vi "WS1050 VPI Test.vi"(0 "Ke2000 Input":refnum<visa-resource-name>, 1 "AD7747 In":refnum<visa-resource-name>, 3 "RFFE In":refnum<visa-resource-name>, 4 "Command":string[](array[string])=["074100", "07413B", "07423B", "07433B", "07413B", "074100"], 5 "CP Control":string, 7 "error out":errorcluster, 8 "Sequence Names":string[](array[string])=["CMin_35V", "C1L_35V", "C2L_35V", "C3L_35V", "ALL_ON_35V", "ALL_OFF_35V"], 9 "S_ValueC1(pF)":dbl=-4.5642919921875, 11 "S_ValueC3(pF)":dbl=-4.9974111328125, 12 "Delay Cap Meas":u32, 13 "S_ValueC2(pF)":dbl=-4.9191376953125, 14 "Status In":string="Idle.....", 17 "VPI Voltage":string) -> (16 "Data Out":string[](array[string]), 20 "Ke2000 Output":refnum<visa-resource-name>, 21 "AD7747 Out":refnum<visa-resource-name>, 23 "RFFE Out":refnum<visa-resource-name>, 24 "Status":string="Idle.....", 25 "IDD_VPI ON":string="43.552393E+0", 26 "IDD_VPI OFF":string="43.360206E+0", 27 "error out 2":errorcluster)   [LabVIEW 2017]
panel:
  out "Sequence":i32(listbox)=5
  out "CMin2_35V":string[](array[string])=["1.184179E+0", "1.241177E+0", "1.250951E+0"]
  out "Cmax 35V":string[](array[string])=["7.353896E+0", "7.168632E+0", "7.184664E+0"]
  out "C3L_Max 35V":string="7.184664E+0"
  out "C2L_Max 35V":string="7.168632E+0"
  out "C1L_Max 35V":string="7.353896E+0"
  out "CMin_35V":string[](array[string])=["1.183737E+0", "1.240778E+0", "1.250697E+0"]
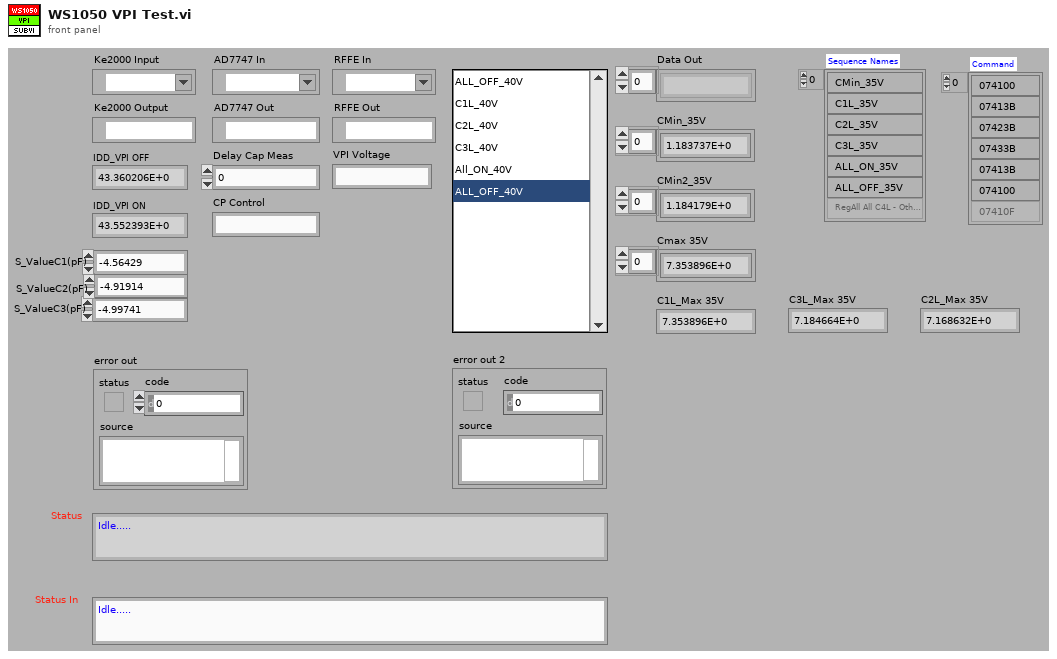
[diagram p1: front panel]
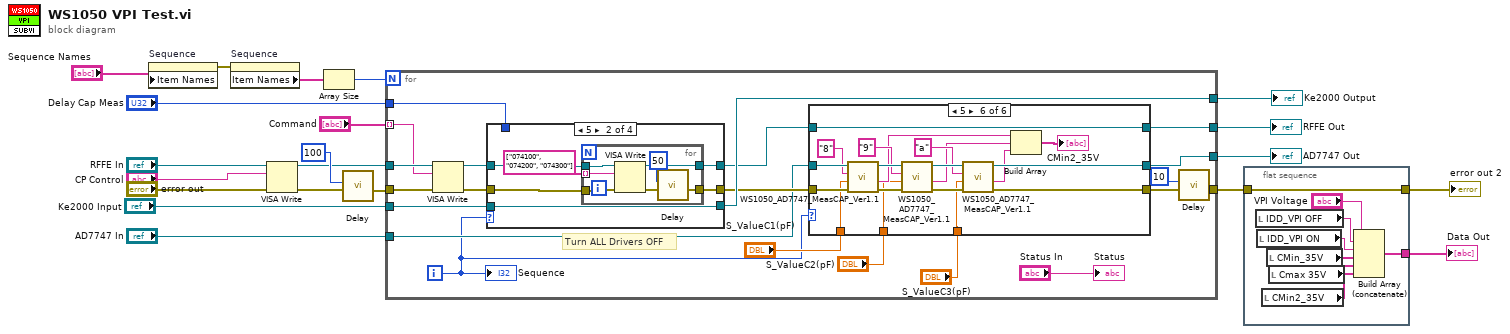
[diagram p0: block diagram]
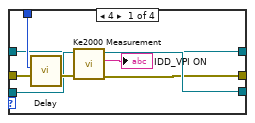
[diagram p2: hidden frame]
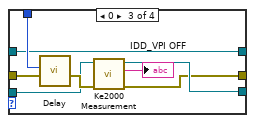
[diagram p3: hidden frame]
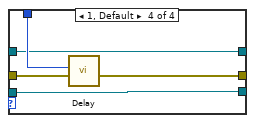
[diagram p4: hidden frame]
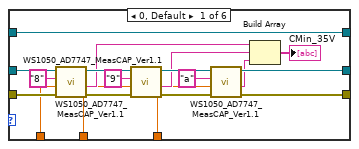
[diagram p5: hidden frame]
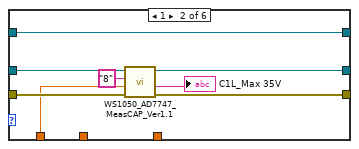
[diagram p6: hidden frame]
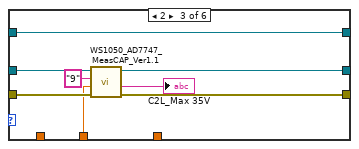
[diagram p7: hidden frame]
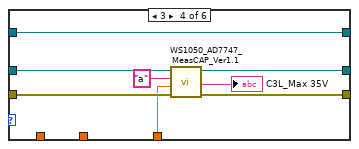
[diagram p8: hidden frame]
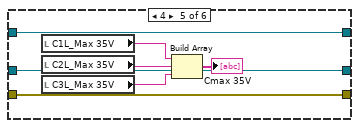
[diagram p9: hidden frame]
diagram:
  n1 = property on="Sequence" class="LstBox (strict)"("Item Names"="Sequence Names") -> (error out=w16:errorcluster)  [unwired: 2 in, 1 out]
  n2 = property on="Sequence" class="LstBox (strict)"(error in=w16) -> ("Item Names"=w14:string[])  [unwired: 1 in, 2 out]
  n3 = VISA Write(VISA resource name="RFFE In", write buffer="CP Control", error in (no error)="error out") -> (VISA resource name out=w11:refnum<visa-resource-name>, error out=w1:errorcluster)  [unwired: 1 out]
  n4 = Array Size(array=w14) -> (size(s)=w17:i32)
  n5 = call "Delay.vi"("error in (no error)"=w1, "milliseconds to wait"=u32 100) -> ("error out"=w2:errorcluster)  [unwired: 9 in]
  n6 = for {
    N: w17 -> [_]
    tunnel: [w28] -> w10
    tunnel: [w34] -> w5
    tunnel: "Delay Cap Meas" -> [w42]
    tunnel: w2 -> [w38]
    tunnel: "Ke2000 Input" -> [w41]
    tunnel: w11 -> [w40]
    tunnel: "Command" -> [w39] mode=indexing
    tunnel: [w36] -> w9
    tunnel: "AD7747 In" -> [w32]
    tunnel: [w30] -> w6
    i -> [w23]
    # "Turn ALL Drivers OFF"
    n7 = VISA Write(VISA resource name=w40, write buffer=w39, error in (no error)=w38) -> (VISA resource name out=w35:refnum<visa-resource-name>, error out=w37:errorcluster)  [unwired: 1 out]
    n8 = case shown="5" w23 {
      tunnel: [w44 w55 w65 w76] -> w33
      tunnel: w42 -> [w46 _ w67 w75]
      tunnel: [w49 w51 w70 w73] -> w36
      tunnel: w37 -> [w47 w56 w68 w74]
      tunnel: w41 -> [w45 w51 w66 w73]
      tunnel: w35 -> [w43 w53 w64 w72]
      tunnel: [w43 w52 w64 w72] -> w31
      frame 4 {
        n9 = call "Delay.vi"("error in (no error)"=w47, "milliseconds to wait"=w46) -> ("error out"=w48:errorcluster)  [unwired: 9 in]
        n10 = call "Ke2000 Measurement.vi"("error in (no error)"=w48, "VISA resource name"=w45) -> ("error out"=w44:errorcluster, "Meas in micro"=→"IDD_VPI ON":string, "VISA resource name out"=w49:refnum<visa-resource-name>)  [unwired: 4 in, 3 out]
      }
      frame 5 {
        n11 = for {
          tunnel: w56 -> [w63]
          tunnel: [w60] -> w55
          tunnel: [w59] -> w52
          tunnel: w53 -> [w58]
          tunnel: string[] ["074100", "074200", "074300"] -> [w57] mode=indexing
          n12 = VISA Write(VISA resource name=w58, write buffer=w57, error in (no error)=w63) -> (VISA resource name out=w59:refnum<visa-resource-name>, error out=w62:errorcluster)  [unwired: 1 out]
          n13 = call "Delay.vi"("error in (no error)"=w62, "milliseconds to wait"=u32 50) -> ("error out"=w60:errorcluster)  [unwired: 9 in]
        }
      }
      frame 0 {
        n14 = call "Delay.vi"("error in (no error)"=w68, "milliseconds to wait"=w67) -> ("error out"=w69:errorcluster)  [unwired: 9 in]
        n15 = call "Ke2000 Measurement.vi"("error in (no error)"=w69, "VISA resource name"=w66) -> ("error out"=w65:errorcluster, "Meas in micro"=→"IDD_VPI OFF":string, "VISA resource name out"=w70:refnum<visa-resource-name>)  [unwired: 4 in, 3 out]
      }
      frame 1, Default {
        n16 = call "Delay.vi"("error in (no error)"=w74, "milliseconds to wait"=w75) -> ("error out"=w76:errorcluster)  [unwired: 9 in]
      }
    }
    n17 = case shown="5" w23 {
      tunnel: w32 -> [w94 w100 w108 w116 w126 w144]
      tunnel: [w85 w102 w110 w118 w125 w135] -> w29
      tunnel: w33 -> [w92 w103 w111 w119 w125 w142]
      tunnel: [w84 w99 w107 w115 w126 w136] -> w34
      tunnel: w31 -> [w80 w97 w105 w113 w124 w130]
      tunnel: [w80 w97 w105 w113 w124 w130] -> w30
      tunnel: "S_ValueC1(pF)" -> [w79 w96 _ _ _ w129]
      tunnel: "S_ValueC2(pF)" -> [w78 _ w104 _ _ w128]
      tunnel: "S_ValueC3(pF)" -> [w77 _ _ w112 _ w127]
      frame 0, Default {
        n18 = call "WS1050_AD7747_MeasCAP_Ver1.1.vi"("error in (no error)"=w92, "OFFSet Cal"=w79, "AD7747_Number"="8", "Control"=w94) -> ("error"=w95:errorcluster, "CAP (pF)"=w83:string, "Control out"=w93:refnum<visa-resource-name>)  [unwired: 3 in, 2 out]
        n19 = call "WS1050_AD7747_MeasCAP_Ver1.1.vi"("error in (no error)"=w95, "OFFSet Cal"=w78, "AD7747_Number"="9", "Control"=w93) -> ("error"=w91:errorcluster, "CAP (pF)"=w82:string, "Control out"=w89:refnum<visa-resource-name>)  [unwired: 3 in, 2 out]
        n20 = call "WS1050_AD7747_MeasCAP_Ver1.1.vi"("error in (no error)"=w91, "OFFSet Cal"=w77, "AD7747_Number"="a", "Control"=w89) -> ("error"=w85:errorcluster, "CAP (pF)"=w81:string, "Control out"=w84:refnum<visa-resource-name>)  [unwired: 3 in, 2 out]
        n21 = Build Array(w83, w82, w81) -> (→"CMin_35V":string[])
      }
      frame 1 {
        n22 = call "WS1050_AD7747_MeasCAP_Ver1.1.vi"("error in (no error)"=w103, "OFFSet Cal"=w96, "AD7747_Number"="8", "Control"=w100) -> ("error"=w102:errorcluster, "CAP (pF)"=→"C1L_Max 35V":string, "Control out"=w99:refnum<visa-resource-name>)  [unwired: 3 in, 2 out]
      }
      frame 2 {
        n23 = call "WS1050_AD7747_MeasCAP_Ver1.1.vi"("error in (no error)"=w111, "OFFSet Cal"=w104, "AD7747_Number"="9", "Control"=w108) -> ("error"=w110:errorcluster, "CAP (pF)"=→"C2L_Max 35V":string, "Control out"=w107:refnum<visa-resource-name>)  [unwired: 3 in, 2 out]
      }
      frame 3 {
        n24 = call "WS1050_AD7747_MeasCAP_Ver1.1.vi"("error in (no error)"=w119, "OFFSet Cal"=w112, "AD7747_Number"="a", "Control"=w116) -> ("error"=w118:errorcluster, "CAP (pF)"=→"C3L_Max 35V":string, "Control out"=w115:refnum<visa-resource-name>)  [unwired: 3 in, 2 out]
      }
      frame 4 {
        n25 = local read "C1L_Max 35V"() -> (w123:string)
        n26 = local read "C2L_Max 35V"() -> (w122:string)
        n27 = local read "C3L_Max 35V"() -> (w121:string)
        n28 = Build Array(w123, w122, w121) -> (→"Cmax 35V":string[])
      }
      frame 5 {
        n29 = call "WS1050_AD7747_MeasCAP_Ver1.1.vi"("error in (no error)"=w142, "OFFSet Cal"=w129, "AD7747_Number"="8", "Control"=w144) -> ("error"=w145:errorcluster, "CAP (pF)"=w133:string, "Control out"=w143:refnum<visa-resource-name>)  [unwired: 3 in, 2 out]
        n30 = call "WS1050_AD7747_MeasCAP_Ver1.1.vi"("error in (no error)"=w145, "OFFSet Cal"=w128, "AD7747_Number"="9", "Control"=w143) -> ("error"=w141:errorcluster, "CAP (pF)"=w132:string, "Control out"=w139:refnum<visa-resource-name>)  [unwired: 3 in, 2 out]
        n31 = call "WS1050_AD7747_MeasCAP_Ver1.1.vi"("error in (no error)"=w141, "OFFSet Cal"=w127, "AD7747_Number"="a", "Control"=w139) -> ("error"=w135:errorcluster, "CAP (pF)"=w131:string, "Control out"=w136:refnum<visa-resource-name>)  [unwired: 3 in, 2 out]
        n32 = Build Array(w133, w132, w131) -> (→"CMin2_35V":string[])
      }
    }
    n33 = call "Delay.vi"("error in (no error)"=w29, "milliseconds to wait"=u32 10) -> ("error out"=w28:errorcluster)  [unwired: 9 in]
    "Sequence" <- w23
    "Status" <- "Status In"
  }
  "Ke2000 Output" <- w9
  "RFFE Out" <- w6
  "AD7747 Out" <- w5
  n34 = flat-sequence {
    tunnel: w10 -> [w148]
    tunnel: [w148] -> w7
    tunnel: [w147] -> w8
    frame #0 {
      n35 = local read "IDD_VPI OFF"() -> (w151:string)
      n36 = local read "IDD_VPI ON"() -> (w150:string)
      n37 = local read "CMin2_35V"() -> (w153:string[])
      n38 = local read "CMin_35V"() -> (w149:string[])
      n39 = local read "Cmax 35V"() -> (w152:string[])
      n40 = Build Array (concatenate)("VPI Voltage", w151, w150, w149, w152, w153) -> (w147:string[])
    }
  }
  "Data Out" <- w8
  "error out 2" <- w7
